vi "String To Number(I64)_csm.vi"(5 "String":string) -> (0 "Numeric":u64)   [LabVIEW 2017, in "API String Arguments Support.lvlib"]
doc: "Converts a string to a 64-bit integer. Supports multiple numeric formats, including standard integer, decimal, hexadecimal, binary, octal, and suffix notations. Returns 0 if conversion fails.\n\n-- <b>Controls</b> --\n- <b>String</b>: Input string.\n\n-- <b>Indicators</b> --\n- <b>Numeric</b>: Converted 64-bit integer."
uses:
  API String Arguments Support.lvlib
  35e04dae-fb20-45f2-b6e6-a1e99b0bae27.vi
  c7c8f582-3164-4c23-83d8-8f64db7f198b.vi
  <userlib>/_NEVSTOP/Communicable State Machine(CSM)/_Shared/CSM Shared.lvlib
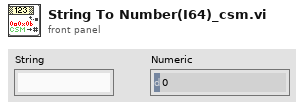
[diagram p1: front panel]
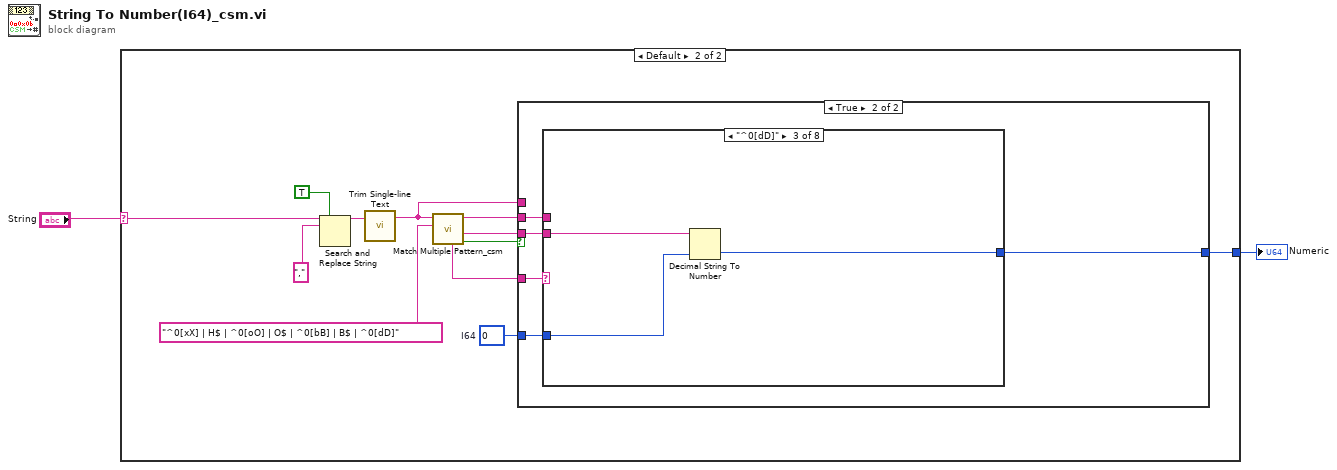
[diagram p0: block diagram]
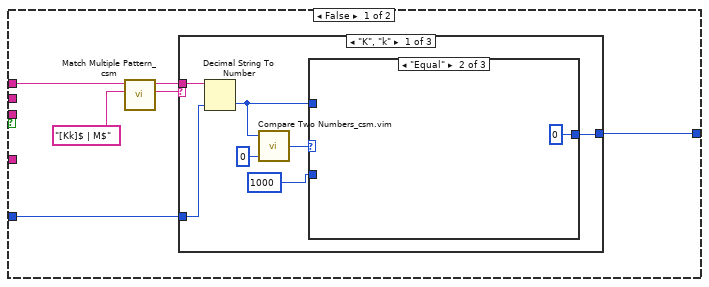
[diagram p3: hidden frame]
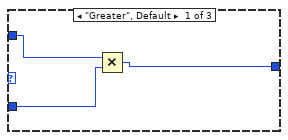
[diagram p4: hidden frame]
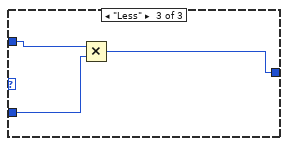
[diagram p5: hidden frame]
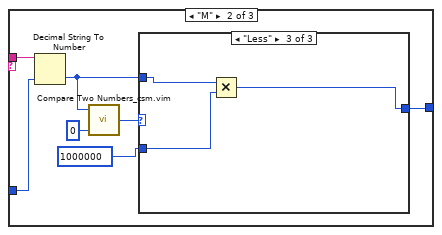
[diagram p6: hidden frame]
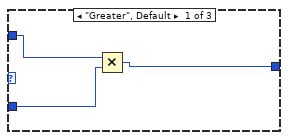
[diagram p7: hidden frame]
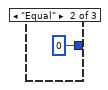
[diagram p8: hidden frame]
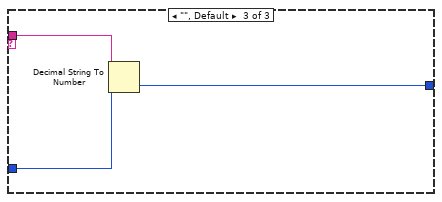
[diagram p9: hidden frame]
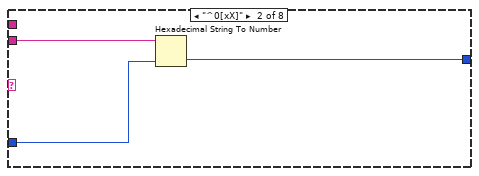
[diagram p11: hidden frame]
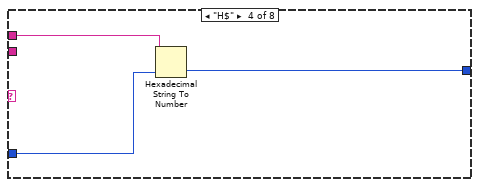
[diagram p12: hidden frame]
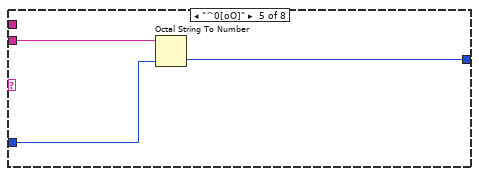
[diagram p13: hidden frame]
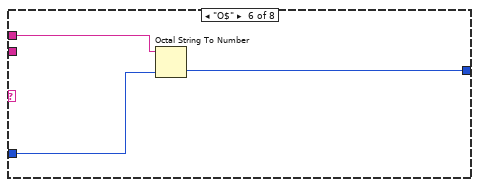
[diagram p14: hidden frame]
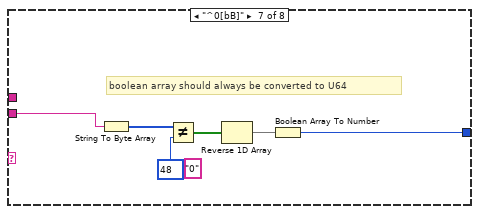
[diagram p15: hidden frame]
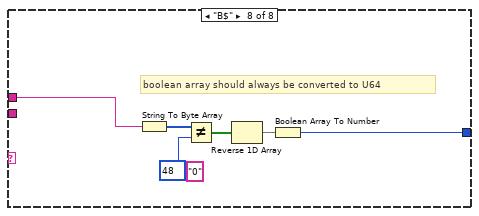
[diagram p16: hidden frame]
diagram:
  n1 = case shown="Default" "String" {
    selector: "String" -> [_ w14]
    tunnel: [_ w5] -> w1
    frame "" {
    }
    frame Default {
      w3 = i64 0  # I64
      n2 = Search and Replace String(replace all?=TRUE ("replace all? (F)"), input string=w14, search string=",") -> (result string=w11:string)  [unwired: 5 in, 3 out]
      n3 = call <userlib>:"Trim Single-line Text.vi"("single-line text"=w11) -> ("trimed text"=w4:string)  [unwired: 2 in]
      n4 = call "Match Multiple Pattern_csm.vi"("regular expression"="^0[xX] | H$ | ^0[oO] | O$ | ^0[bB] | B$ | ^0[dD]", "string"=w4) -> ("Found?"=w9:bool, "after substring"=w7:string, "before substring"=w6:string, "pattern matched"=w8:string)  [unwired: 5 in, 1 out]
      n5 = case shown="True" w9 {
        tunnel: w8 -> [_ w56]
        tunnel: w7 -> [_ w55]
        tunnel: w6 -> [_ w54]
        tunnel: [w15 w53] -> w5
        tunnel: w4 -> [w16 _]
        tunnel: w3 -> [w17 w52]
        frame False {
          n6 = call "Match Multiple Pattern_csm.vi"("regular expression"="[Kk]$ | M$", "string"=w16) -> ("match substring"=w19:string, "before substring"=w18:string)  [unwired: 5 in, 3 out]
          n7 = case shown="\"K\", \"k\"" w19 {
            tunnel: [w24 w38 w51] -> w15
            tunnel: w17 -> [w23 w37 w50]
            tunnel: w18 -> [w27 w41 w49]
            frame "K", "k" {
              n8 = Decimal String To Number(string=w27, default (0L)=w23) -> (number=w22:i64)  [unwired: 1 in, 1 out]
              n9 = call "Compare Two Numbers_csm.vim"("Ref"=0, "Number"=w22) -> ("Result"=w25:enum16{"Greater", "Equal", "Less"})  [unwired: 1 in, 2 out]
              n10 = case shown="\"Equal\"" w25 {
                tunnel: [w30 i64 0 w34] -> w24
                tunnel: w22 -> [w29 _ w33]
                tunnel: i64 1000 ("y") -> [w28 _ w32]
                frame "Greater", Default {
                  n11 = Multiply(x=w29, y=w28) -> (x*y=w30:i64)
                }
                frame "Equal" {
                }
                frame "Less" {
                  n12 = Multiply(x=w33, y=w32) -> (x*y=w34:i64)
                }
              }
            }
            frame "M" {
              n13 = Decimal String To Number(string=w41, default (0L)=w37) -> (number=w36:i64)  [unwired: 1 in, 1 out]
              n14 = call "Compare Two Numbers_csm.vim"("Ref"=0, "Number"=w36) -> ("Result"=w39:enum16{"Greater", "Equal", "Less"})  [unwired: 1 in, 2 out]
              n15 = case shown="\"Less\"" w39 {
                tunnel: [w44 i64 0 w48] -> w38
                tunnel: w36 -> [w43 _ w47]
                tunnel: i64 1000000 ("y") -> [w42 _ w46]
                frame "Greater", Default {
                  n16 = Multiply(x=w43, y=w42) -> (x*y=w44:i64)
                }
                frame "Equal" {
                }
                frame "Less" {
                  n17 = Multiply(x=w47, y=w46) -> (x*y=w48:i64)
                }
              }
            }
            frame "", Default {
              n18 = Decimal String To Number(string=w49, default (0L)=w50) -> (number=w51:i64)  [unwired: 1 in, 1 out]
            }
          }
        }
        frame True {
          n19 = case shown="\"^0[dD]\"" w56 {
            tunnel: w55 -> [_ w60 w63 _ w69 _ w77 _]
            tunnel: w54 -> [_ _ _ w65 _ w71 _ w81]
            tunnel: [w57 w59 w62 w66 w68 w72 w78 w84] -> w53
            tunnel: w52 -> [w57 w58 w61 w64 w67 w70 _ _]
            frame Default {
            }
            frame "^0[xX]" {
              n20 = Hexadecimal String To Number(string=w60, default (0uL)=w58) -> (number=w59:i64)  [unwired: 1 in, 1 out]
            }
            frame "^0[dD]" {
              n21 = Decimal String To Number(string=w63, default (0L)=w61) -> (number=w62:i64)  [unwired: 1 in, 1 out]
            }
            frame "H$" {
              n22 = Hexadecimal String To Number(string=w65, default (0uL)=w64) -> (number=w66:i64)  [unwired: 1 in, 1 out]
            }
            frame "^0[oO]" {
              n23 = Octal String To Number(2:w67, 4:w69) -> (0:w68:i64)  [unwired: 1 in, 1 out]
            }
            frame "O$" {
              n24 = Octal String To Number(2:w70, 4:w71) -> (0:w72:i64)  [unwired: 1 in, 1 out]
            }
            frame "^0[bB]" {
              (unwired) "0" ("search string")
              # "boolean array should always be converted to U64"
              n25 = String To Byte Array(string=w77) -> (unsigned byte array=w76:u8[])
              n26 = Not Equal?(x=w76, y=u8 48) -> (x != y?=w74:bool[])
              n27 = Reverse 1D Array(array=w74) -> (reversed array=w73:bool[])
              n28 = Boolean Array To Number(Boolean array=w73) -> (number=w78:u64)
            }
            frame "B$" {
              (unwired) "0" ("search string")
              # "boolean array should always be converted to U64"
              n29 = String To Byte Array(string=w81) -> (unsigned byte array=w83:u8[])
              n30 = Not Equal?(x=w83, y=u8 48) -> (x != y?=w82:bool[])
              n31 = Reverse 1D Array(array=w82) -> (reversed array=w80:bool[])
              n32 = Boolean Array To Number(Boolean array=w80) -> (number=w84:u64)
            }
          }
        }
      }
    }
  }
  "Numeric" <- w1
